vi "I2C LCD Raw ADC.vi"() -> ()   [LabVIEW 2023, in "CTI-Visa-Scratchpad.lvlib"]
uses:
  CTI-Visa-Scratchpad.lvlib
  CTI-Visa-DeviceLib/LCD-I2C/LCD Size.ctl
  CTI-Visa/I2C Options.ctl
  CTI-Visa-DeviceLib/LCD-I2C/Position.ctl
  CTI-Visa-DeviceLib/LCD-I2C/LCD-I2C.lvclass
  CTI-Visa/CTI-Visa.lvlib
  <vilib>/ptbypt/NI_PtbyPt.lvlib
panel:
  out "Rate":dbl format="%0.2f"
  out "Value":u16
  in  "ADC":i32
  in  "Address":u8=39 format="%.0x"
  in  "I2C Options":T1={"Bus"=0, "Baud"=400000, "SCL GPIO"=16, "SDA GPIO"=17}
  in  "LCD Size":T2={"Rows"=2, "Cols"=16}
  in  "stop":bool
  out "error out":errorcluster
  in  "Port":refnum<visa-resource-name>="COM4"
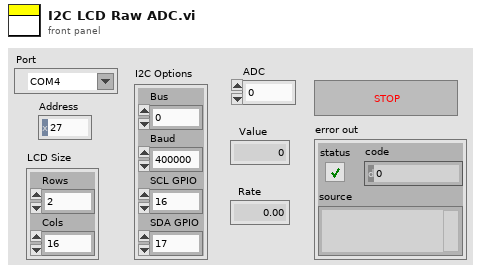
[diagram p1: front panel]
types:
  T1 = typedef "CTI-Visa.lvlib/I2C Options.ctl" = cluster{"Bus":u8, "Baud":u32, "SCL GPIO":i32, "SDA GPIO":i32}
  T2 = typedef "CTI-Visa-DeviceLib.lvlib/LCD-I2C.lvclass/LCD Size.ctl" = cluster{"Rows":u8, "Cols":u8}
  T3 = typedef "CTI-Visa-DeviceLib.lvlib/LCD-I2C.lvclass/Position.ctl" = cluster{"Row":u8, "Col":u8}
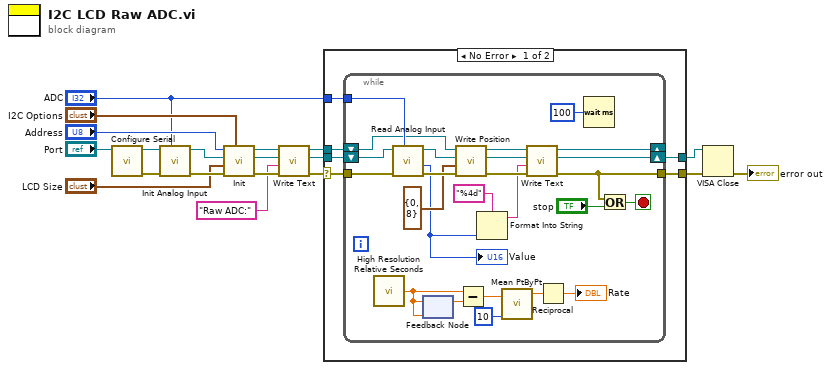
[diagram p0: block diagram]
diagram:
  n1 = call "Configure Serial.vi"("VISA resource name in"="Port") -> ("error out"=w10:errorcluster, "VISA resource name"=w11:refnum<visa-resource-name>)  [unwired: 9 in]
  n2 = call "Init Analog Input.vi"("ADC"="ADC", "error in (no error)"=w10, "VISA resource name in"=w11) -> ("error out"=w19:errorcluster, "VISA resource name"=w2:refnum<visa-resource-name>)  [unwired: 7 in]
  n3 = call "Init.vi"("I2C Options"="I2C Options", "error in (no error)"=w19, "LCD Size"="LCD Size", "VISA resource name in"=w2, "Address"="Address") -> ("error out"=w14:errorcluster, "VISA resource name"=w5:refnum<visa-resource-name>, "LCD-I2C out"=w7:refnum<class "LCD-I2C.lvclass">)  [unwired: 4 in]
  n4 = call "Write Text.vi"("error in (no error)"=w14, "Text"="Raw ADC:", "VISA resource name in"=w5, "LCD-I2C in"=w7) -> ("error out"=w8:errorcluster, "VISA resource name"=w4:refnum<visa-resource-name>, "LCD-I2C out"=w6:refnum<class "LCD-I2C.lvclass">)  [unwired: 5 in]
  n5 = case shown="No Error" w8 {
    selector: w8 -> [w23 w52]
    tunnel: w4 -> [w24 w51]
    tunnel: w6 -> [w25 _]
    tunnel: [w20 w52] -> w13
    tunnel: [w22 w51] -> w12
    tunnel: "ADC" -> [w21 _]
    frame No Error {
      n6 = while {
        shift-right: [w36] -> _
        shift-left: w25 -> [w46]
        shift-right: [w37] -> w22
        shift-left: w24 -> [w49]
        tunnel: w23 -> [w48]
        tunnel: w21 -> [w47]
        tunnel: [w38] -> w20
        stop <- w50 stop-if-true
        n7 = call <vilib>:"High Resolution Relative Seconds.vi"() -> ("relative seconds"=w31:dbl)
        n8 = call "Read Analog Input.vi"("ADC"=w47, "error in (no error)"=w48, "VISA resource name in"=w49) -> ("error out"=w44:errorcluster, "Value"=w34:u16, "VISA resource name"=w45:refnum<visa-resource-name>)  [unwired: 6 in]
        "Value" <- w34
        n9 = feedback-in #1(w31) -> ()
        n10 = feedback #1(w31) -> (w30:dbl)
        n11 = call "Write Position.vi"("error in (no error)"=w44, "Position"=T3 {"Row"=0, "Col"=8}, "VISA resource name in"=w45, "LCD-I2C in"=w46) -> ("error out"=w39:errorcluster, "VISA resource name"=w40:refnum<visa-resource-name>, "LCD-I2C out"=w41:refnum<class "LCD-I2C.lvclass">)  [unwired: 5 in]
        n12 = Subtract(x=w31, y=w30) -> (x-y=w29:dbl)
        n13 = Format Into String(format string="%4d", w34) -> (resulting string=w33:string)  [unwired: 2 in, 1 out]
        n14 = call <vilib>:"Mean PtByPt.vi"("x"=w29, "sample length"=10) -> ("mean"=w27:dbl)  [unwired: 2 in, 1 out]
        n15 = call "Write Text.vi"("error in (no error)"=w39, "Text"=w33, "VISA resource name in"=w40, "LCD-I2C in"=w41) -> ("error out"=w38:errorcluster, "VISA resource name"=w37:refnum<visa-resource-name>, "LCD-I2C out"=w36:refnum<class "LCD-I2C.lvclass">)  [unwired: 5 in]
        n16 = Reciprocal(x=w27) -> (1/x=→"Rate":dbl)
        n17 = Wait (ms)(milliseconds to wait=u32 100) -> ()  [unwired: 1 out]
        n18 = Or(x=w38, y="stop") -> (x .or. y?=w50:bool)
      }
    }
    frame Error {
    }
  }
  n19 = VISA Close(VISA resource name=w12, error in (no error)=w13) -> (error out=→"error out":errorcluster)
